vi "step1 SolveUpperCross.vi"(8 "error in (no error)":errorcluster, 11 "cube in":T1) -> (0 "error out":errorcluster, 1 "upper cross solved?":bool, 3 "cube out":T1)   [LabVIEW 2011]
doc: "Rotate cube as necessary so that the top middle piece matches the desired start colour.\n\nNo transformations are done in this VI, the operations are loaded on the the operation queue bus."
uses:
  Typedef/cube.ctl
  Typedef/face.ctl
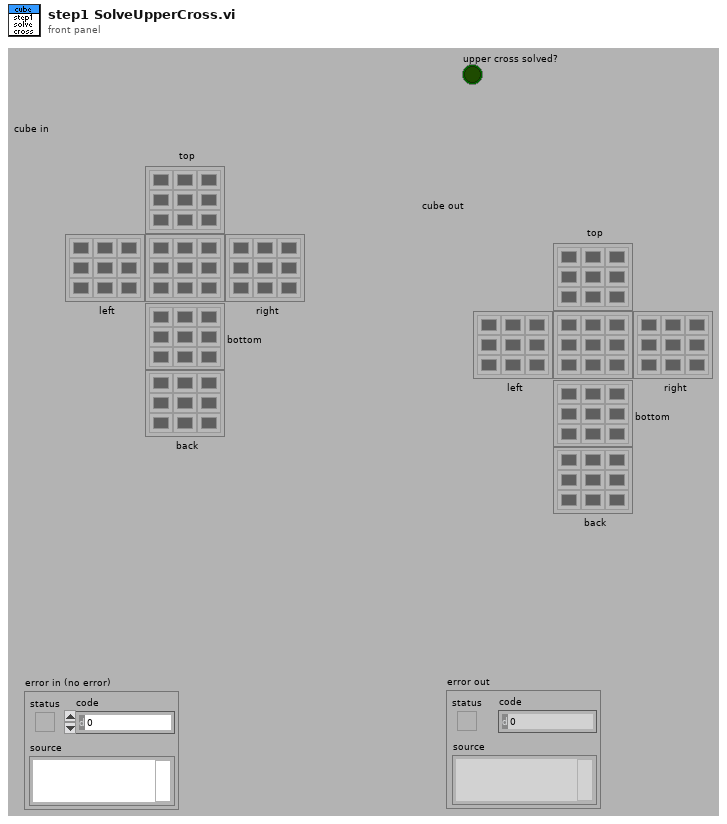
[diagram p1: front panel]
types:
  T1 = typedef "cube.ctl" = cluster{"top":T2, "left":T2, "right":T2, "bottom":T2, "back":T2, "front":T2}
  T2 = typedef "face.ctl" = u32[][]
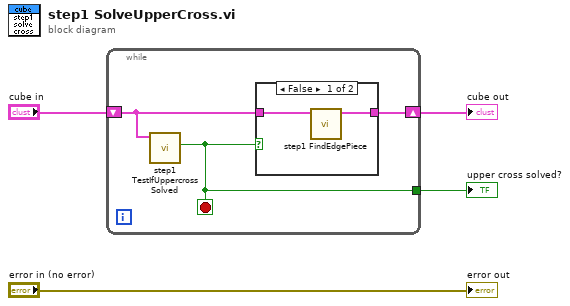
[diagram p0: block diagram]
diagram:
  n1 = while {
    shift-right: [w6] -> w1
    shift-left: "cube in" -> [w7]
    tunnel: [w5] -> w2
    stop <- w5 stop-if-true
    n2 = call "step1 TestIfUppercrossSolved.vi"("cube in"=w7) -> ("uppercross solved?"=w5:bool)  [unwired: 9 in, 1 out]
    n3 = case shown="False" w5 {
      tunnel: w7 -> [w9 w10]
      tunnel: [w8 w10] -> w6
      frame False {
        n4 = call "step1 FindEdgePiece.vi"("cube in"=w9) -> ("cube out"=w8:T1)  [unwired: 9 in, 1 out]
      }
      frame True {
      }
    }
  }
  "upper cross solved?" <- w2
  "cube out" <- w1
  "error out" <- "error in (no error)"
